vi "advTDMScontents.vi"(1 "file path":path) -> (0 "TDMS contents":cluster{string, string[]}[](array[cluster]))   [LabVIEW 2013]
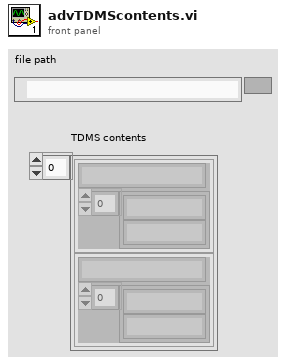
[diagram p1: front panel]
types:
  T1 = enum16{"open", "open or create", "create or replace", "create", "open (read-only)"}
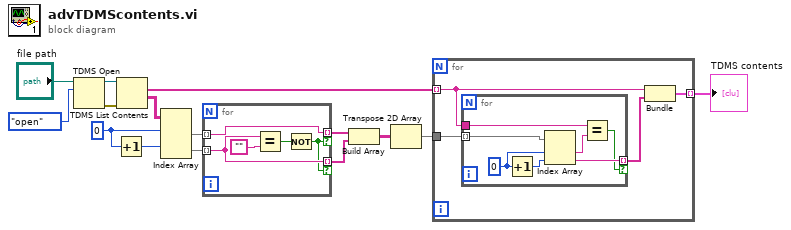
[diagram p0: block diagram]
diagram:
  w10 = 0
  n1 = TDMS Open(10:T1."open" ("operation (0:open)"), 11:"file path") -> (0:w12:errorcluster, 3:w13:refnum<k34>)  [unwired: 5 in]
  n2 = Increment(x=w10) -> (x+1=w8:i32)
  n3 = TDMS List Contents(4:w12, 7:w13) -> (1:w11:string[][], 2:w4:string[])  [unwired: 1 in, 2 out]
  n4 = Index Array(array=w11, index (row) #1=w10, index (row) #2=w8) -> (element #1=w9:string[], element #2=w7:string[])  [unwired: 2 in]
  n5 = for {
    tunnel: w9 -> [w20] mode=indexing
    tunnel: w7 -> [w19] mode=indexing
    tunnel: [w20] -> w6 mode=indexing if=w16
    tunnel: [w19] -> w5 mode=indexing if=w16
    n6 = Equal?(x=w19, y="") -> (x = y?=w17:bool)
    n7 = Not(x=w17) -> (.not. x?=w16:bool)
  }
  n8 = Build Array(w6, w5) -> (w3:string[][])
  n9 = Transpose 2D Array(2D array=w3) -> (transposed array=w2:string[][])
  n10 = for {
    tunnel: w4 -> [w22] mode=indexing
    tunnel: w2 -> [w24]
    tunnel: [w21] -> w1 mode=indexing
    n11 = for {
      tunnel: w22 -> [w31]
      tunnel: w24 -> [w30] mode=indexing
      tunnel: [w26] -> w23 mode=indexing if=w25
      w28 = 0
      n12 = Increment(x=w28) -> (x+1=w29:i32)
      n13 = Index Array(array=w30, index #1=w28, index #2=w29) -> (element #1=w27:string, element #2=w26:string)
      n14 = Equal?(x=w31, y=w27) -> (x = y?=w25:bool)
    }
    n15 = Bundle(w22, w23) -> (w21:cluster{string, string[]})  [unwired: 1 in]
  }
  "TDMS contents" <- w1
